vi "Create.vi"(5 "String Ends With in":refnum<class "String Ends With.lvclass">, 8 "error in (no error)":errorcluster, 11 "Suffix":string) -> (0 "error out":errorcluster, 3 "String Ends With":refnum<class "String Ends With.lvclass">)   [LabVIEW 2017, in "Transparent Assertions.lvlib" / "String Ends With.lvclass"]
uses:
  String Ends With.lvclass
  String Ends With.lvclass/String Ends With.ctl
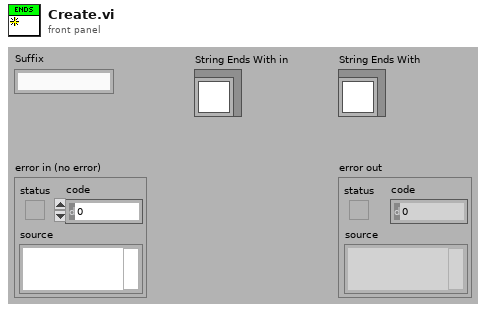
[diagram p1: front panel]
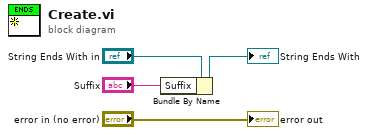
[diagram p0: block diagram]
diagram:
  n1 = Bundle By Name(cluster="String Ends With in", "Suffix"="Suffix") -> (→"String Ends With":refnum<class "String Ends With.lvclass">)
  "error out" <- "error in (no error)"
